vi "Dequeue as String.vi"(6 "timeout in ms (-1)":i32, 8 "error in (no error)":errorcluster, 11 "LVQueue Sink in":refnum<class "LVQueue Sink.lvclass">) -> (0 "error out":errorcluster, 2 "Log Event as String":string, 3 "LVQueue Sink out":refnum<class "LVQueue Sink.lvclass">, 4 "Timed Out?":bool)   [LabVIEW 2018, in "MVA Framework.lvlib" / "LVQueue Sink.lvclass"]
uses:
  LVQueue Sink.lvclass
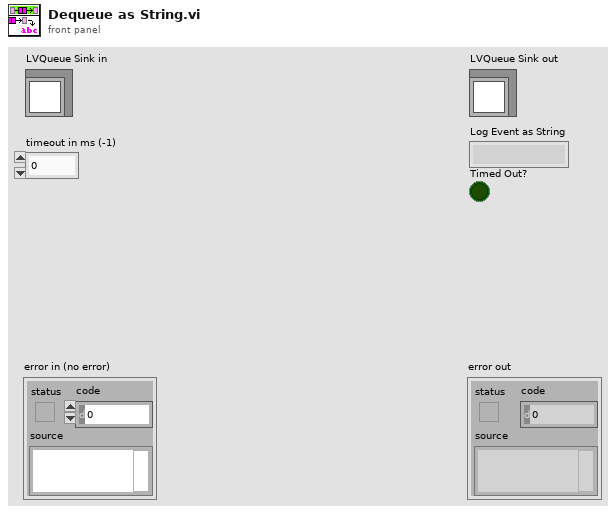
[diagram p1: front panel]
types:
  T1 = typedef "Composed Log.lvlib/Application Logger.lvclass/Log Packet.ctl" = cluster{"Data To Log":string, "Source":string, "Event Level":T2, "Event Time":timestamp}
  T2 = typedef "Composed Log.lvlib/Log Sink.lvclass/Log Level.ctl" = enum16{"Debug", "Info", "Warning", "Error", "Critical"}
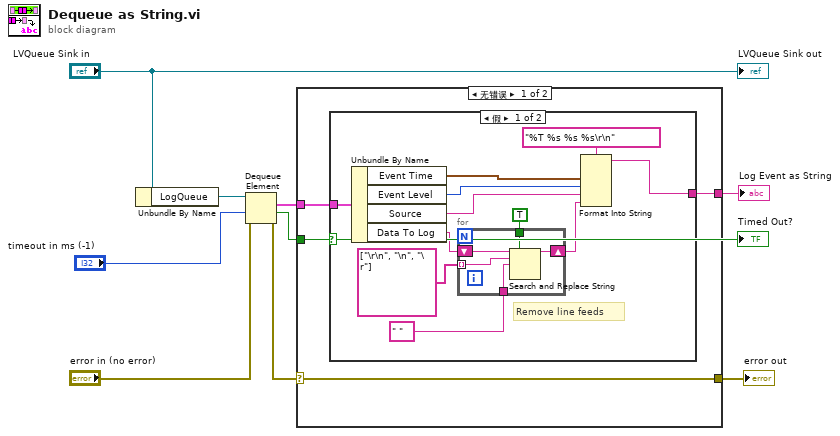
[diagram p0: block diagram]
diagram:
  n1 = Unbundle By Name("LVQueue Sink in") -> ("LogQueue"=w8:refnum<queue>)
  n2 = Dequeue Element(queue=w8, timeout in ms (-1)="timeout in ms (-1)", error in (no error)="error in (no error)") -> (element=w4:T1, timed out?=w5:bool, error out=w2:errorcluster)  [unwired: 1 out]
  "Timed Out?" <- w5
  n3 = case shown="无错误" w2 {
    selector: w2 -> [w10 w30]
    tunnel: w5 -> [w13 _]
    tunnel: w4 -> [w12 _]
    tunnel: [w11 _] -> w3
    tunnel: [w10 w30] -> w1
    frame No Error {
      n4 = case shown="假" w13 {
        tunnel: w12 -> [w15 _]
        tunnel: [w14 _] -> w11
        frame False {
          # "Remove line feeds"
          n5 = Unbundle By Name(w15) -> ("Event Time"=w24:timestamp, "Event Level"=w22:T2, "Source"=w21:string, "Data To Log"=w20:string)
          n6 = for {
            shift-right: [w28] -> w19
            shift-left: w20 -> [w29]
            tunnel: TRUE ("replace all? (F)") -> [w27]
            tunnel: string[] ["\r\n", "\n", "\r"] ("search string") -> [w26] mode=indexing
            tunnel: " " ("replace string (\"\")") -> [w25]
            n7 = Search and Replace String(replace all?=w27, input string=w29, search string=w26, replace string=w25) -> (result string=w28:string)  [unwired: 4 in, 3 out]
          }
          n8 = Format Into String(format string="%T %s %s %s\r\n", w24, w22, w21, w19) -> (resulting string=w14:string)  [unwired: 2 in, 1 out]
        }
        frame True {
        }
      }
    }
    frame Error {
    }
  }
  "error out" <- w1
  "Log Event as String" <- w3
  "LVQueue Sink out" <- "LVQueue Sink in"
